vi "Data_Pull_Zmodifiy_Global.vi"(0 "Ceiling":sgl) -> ()   [LabVIEW 2016]
uses:
  Utility/Global Constants.vi
  Utility/Global_Sensor.vi
  Utility/Global_Stage.vi
  Utility/Global_Array.vi
  Program Files/MicroEpsilon/MEDAQLib-3.2.3.19901/Samples/LabView/MEDAQLib/MEDAQLib.lvlib
panel:
  out "Abort Loop":bool
  out "ValueHandle":dbl[](array[numeric])
  in  "block":i32=1
  in  "maxValue":i32=1
  out "avail":i32
  out "Buffer Error":i32
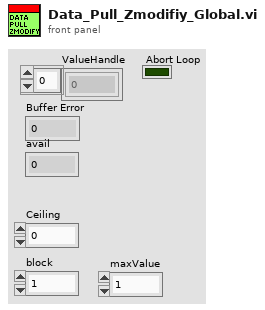
[diagram p1: front panel]
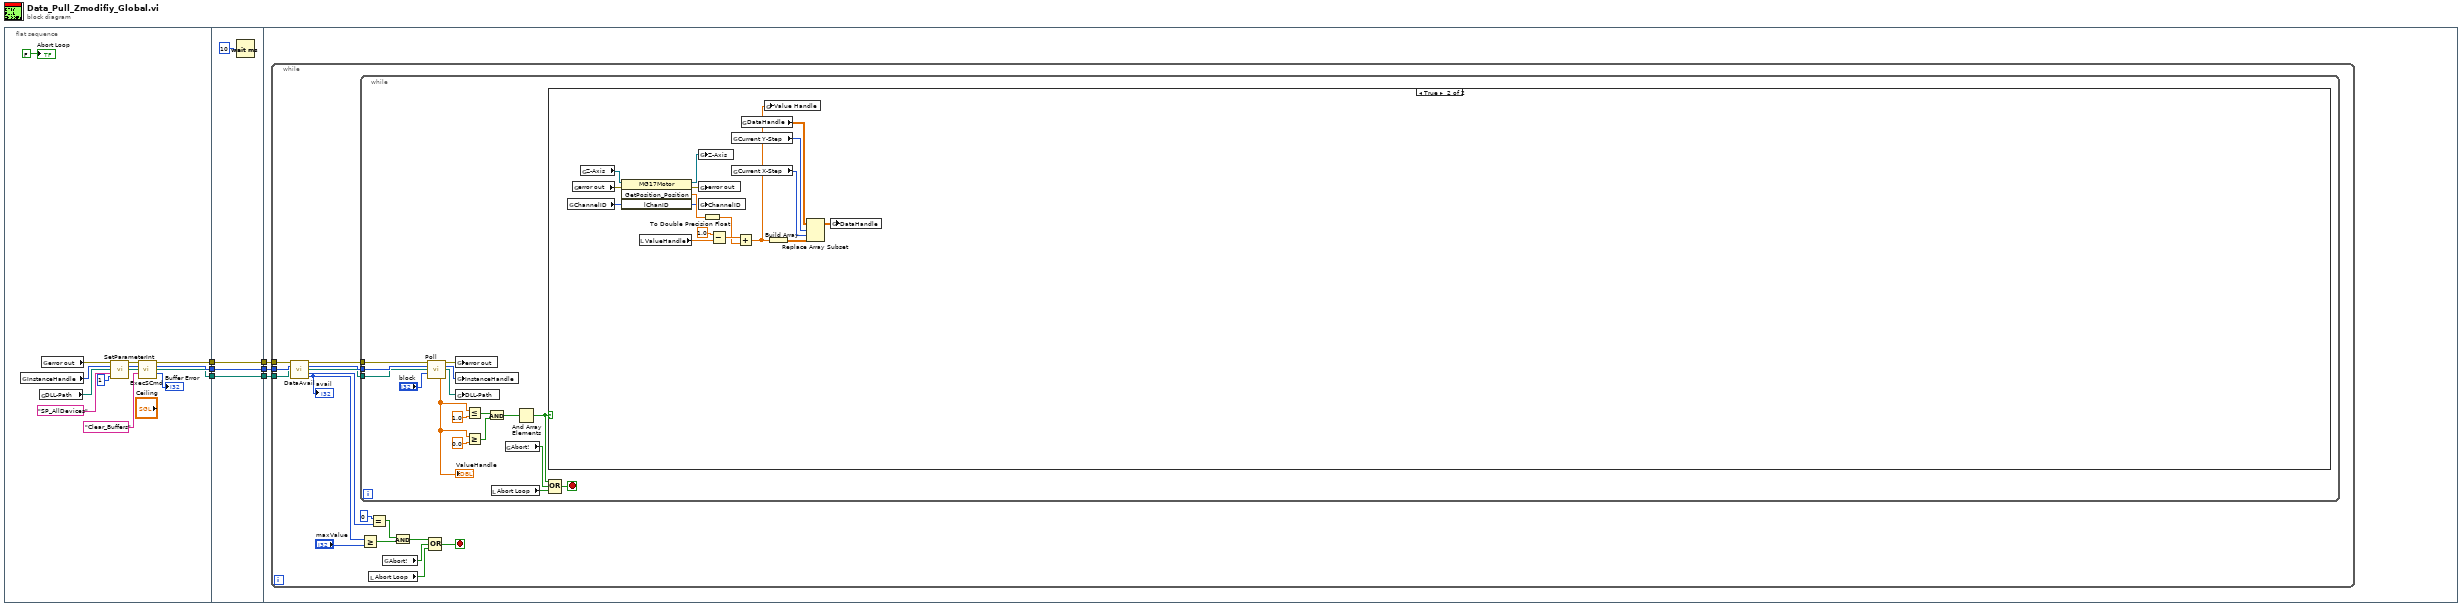
[diagram p0: block diagram]
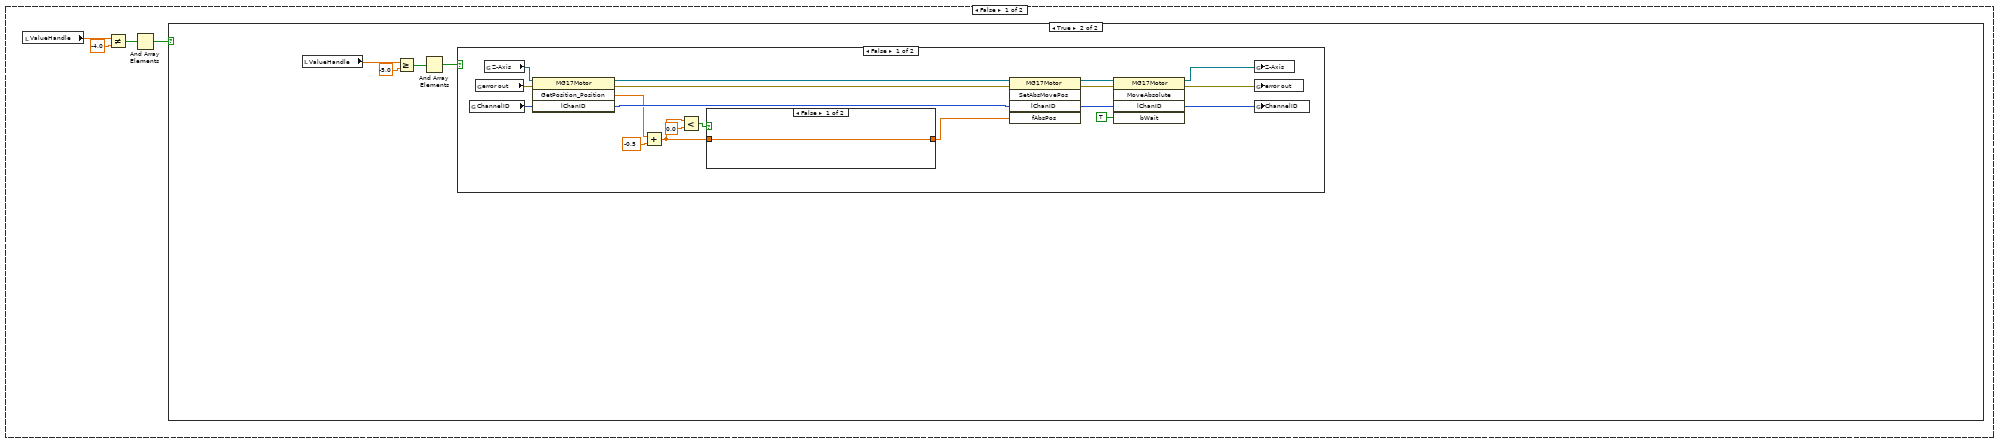
[diagram p2: hidden frame]
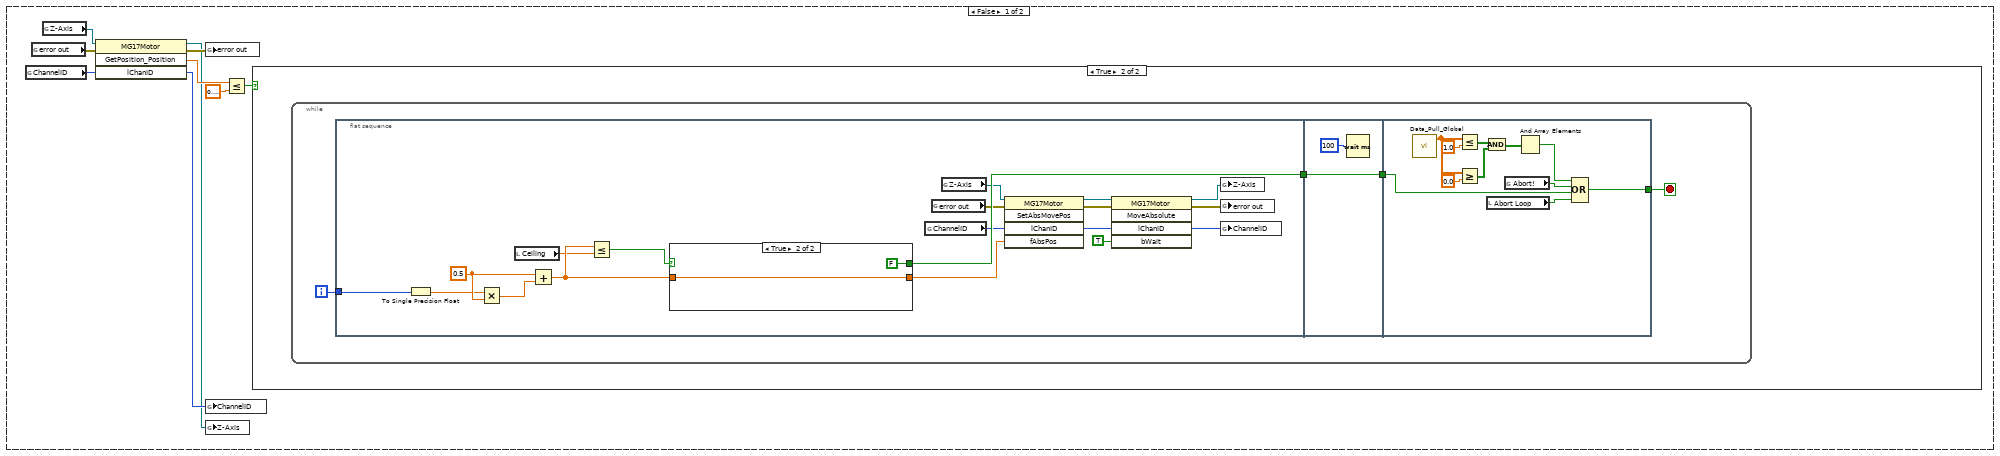
[diagram p3: hidden frame]
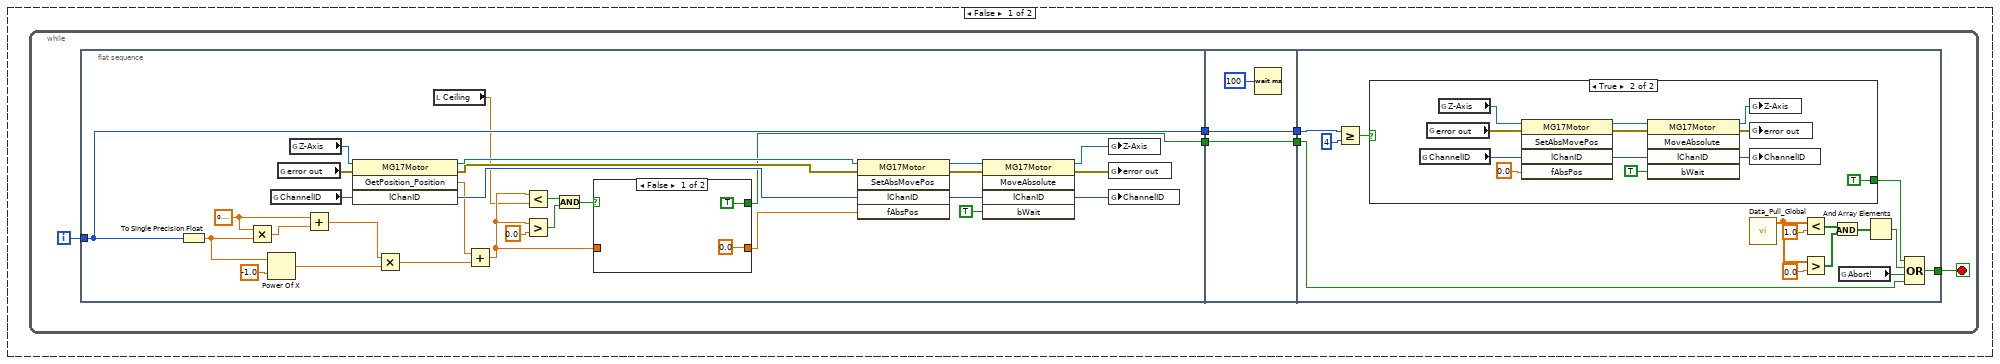
[diagram p4: hidden frame]
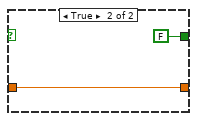
[diagram p5: hidden frame]
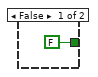
[diagram p6: hidden frame]
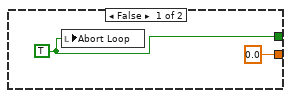
[diagram p7: hidden frame]
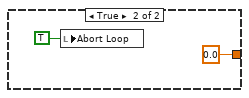
[diagram p8: hidden frame]
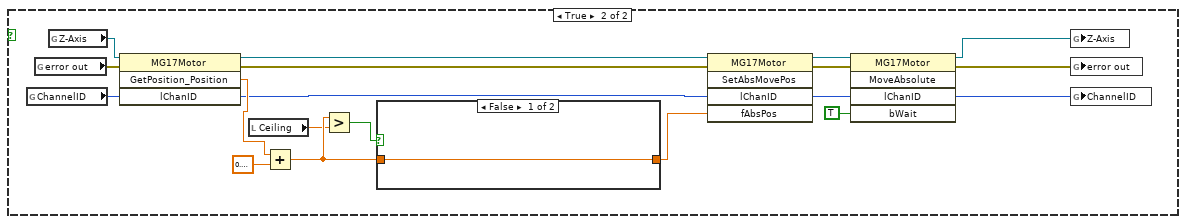
[diagram p9: hidden frame]
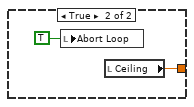
[diagram p10: hidden frame]
diagram:
  n1 = flat-sequence {
    tunnel: [w14] -> w6
    tunnel: [w13] -> w5
    tunnel: [w12] -> w4
    tunnel: [w23] -> w3
    tunnel: w6 -> [w23]
    tunnel: [w22] -> w2
    tunnel: w5 -> [w22]
    tunnel: [w21] -> w1
    tunnel: w4 -> [w21]
    tunnel: w1 -> [w25]
    tunnel: w2 -> [w26]
    tunnel: w3 -> [w27]
    frame #0 {
      n2 = global read "Global_Sensor.vi" "InstanceHandle"() -> (w8:u32)
      n3 = global read "Global_Sensor.vi" "DLL-Path"() -> (w7:path)
      n4 = global read "Global Constants.vi" "error out"() -> (w9:errorcluster)
      n5 = call "SetParameterInt.vi"("Fehler (Eingang, kein Fehler)"=w9, "instanceHandle"=w8, "DLL-Path"=w7, "paramName"="SP_AllDevices", "paramValue"=1) -> ("Fehler (Ausgang)"=w15:errorcluster, "instanceHandle"=w16:u32, "DLL-Path"=w17:path)  [unwired: 7 in, 1 out]
      n6 = call "ExecSCmd.vi"("Fehler (Eingang, kein Fehler)"=w15, "instanceHandle"=w16, "DLL-Path"=w17, "sensorCommand"="Clear_Buffers") -> ("Fehler (Ausgang)"=w14:errorcluster, "instanceHandle"=w13:u32, "DLL-Path"=w12:path, "ERR_CODE"=→"Buffer Error":i32)  [unwired: 8 in]
      "Abort Loop" <- FALSE ("Abort Loop")
    }
    frame #1 {
      n7 = Wait (ms)(milliseconds to wait=u32 10 ("Timer-Wert (ms)")) -> ()  [unwired: 1 out]
    }
    frame #2 {
      n8 = while {
        tunnel: w27 -> [w38]
        tunnel: w26 -> [w37]
        tunnel: w25 -> [w36]
        stop <- w29 stop-if-true
        n9 = call "DataAvail.vi"("Fehler (Eingang, kein Fehler)"=w38, "instanceHandle"=w37, "DLL-Path"=w36) -> ("Fehler (Ausgang)"=w34:errorcluster, "instanceHandle"=w33:u32, "DLL-Path"=w32:path, "ERR_CODE"=w43:i32, "avail"=w41:i32)  [unwired: 8 in]
        "avail" <- w41
        n10 = while {
          tunnel: w34 -> [w59]
          tunnel: w33 -> [w58]
          tunnel: w32 -> [w57]
          stop <- w49 stop-if-true
          n11 = call "Poll.vi"("Fehler (Eingang, kein Fehler)"=w59, "instanceHandle"=w58, "DLL-Path"=w57, "maxValues"="block") -> ("Fehler (Ausgang)"=w47:errorcluster, "instanceHandle"=w45:u32, "DLL-Path"=w44:path, "scaledData"=w51:dbl[])  [unwired: 6 in, 2 out]
          "ValueHandle" <- w51
          n12 = global write "Global Constants.vi" "error out"(w47) -> ()
          n13 = global write "Global_Sensor.vi" "InstanceHandle"(w45) -> ()
          n14 = global write "Global_Sensor.vi" "DLL-Path"(w44) -> ()
          n15 = Less Or Equal?(x=w51, y=1.0 ("Obergrenze")) -> (x <= y?=w54:bool[])
          n16 = Greater Or Equal?(x=w51, y=0.0 ("Untergrenze")) -> (x >= y?=w53:bool[])
          n17 = And(x=w54, y=w53) -> (x .and. y?=w52:bool[])
          n18 = local read "Abort Loop"() -> (w46:bool)
          n19 = global read "Global Constants.vi" "Abort!"() -> (w48:bool)
          n20 = And Array Elements(Boolean array=w52) -> (logical AND=w50:bool)
          n21 = case shown="True" w50 {
            frame False {
              n22 = local read "ValueHandle"() -> (w63:dbl[])
              n23 = Not Equal?(x=w63, y=-4.0) -> (x != y?=w62:bool[])
              n24 = And Array Elements(Boolean array=w62) -> (logical AND=w61:bool)
              n25 = case shown="True" w61 {
                frame False {
                  n26 = global read "Global_Stage.vi" "ChannelID"() -> (w68:i32)
                  n27 = global read "Global Constants.vi" "error out"() -> (w70:errorcluster)
                  n28 = global read "Global_Stage.vi" "Z-Axis"() -> (w66:refnum<k7>)
                  n29 = invoke class="MG17Motor" method="GetPosition_Position"(reference=w66, error in=w70, "lChanID"=w68) -> (reference out=w65:refnum<k7>, error out=w69:errorcluster, "GetPosition_Position"=w71:sgl, "lChanID"=w67:i32)  [unwired: 1 in]
                  n30 = global write "Global Constants.vi" "error out"(w69) -> ()
                  n31 = global write "Global_Stage.vi" "ChannelID"(w67) -> ()
                  n32 = global write "Global_Stage.vi" "Z-Axis"(w65) -> ()
                  n33 = Less Or Equal?(x=w71, y=sgl 0.1) -> (x <= y?=w72:bool)
                  n34 = case shown="True" w72 {
                    frame False {
                      n35 = while {
                        i -> [w79]
                        stop <- w78 stop-if-true
                        n36 = flat-sequence {
                          tunnel: [w88] -> w77
                          tunnel: w79 -> [w87]
                          tunnel: [w87] -> w74
                          tunnel: w77 -> [w115]
                          tunnel: [w115] -> w76
                          tunnel: [w114] -> w75
                          tunnel: w74 -> [w114]
                          tunnel: [w128] -> w78
                          tunnel: w76 -> [w123]
                          tunnel: w75 -> [w122]
                          frame #0 {
                            w105 = sgl 0.4 ("x")
                            n37 = To Single Precision Float(number=w87) -> (single precision float=w106:sgl)
                            n38 = Multiply(x=w105, y=w106) -> (x*y=w104:sgl)
                            n39 = Power Of X(1:sgl -1.0 ("x"), 2:w106) -> (0:w108:sgl)
                            n40 = global read "Global_Stage.vi" "ChannelID"() -> (w81:i32)
                            n41 = global read "Global Constants.vi" "error out"() -> (w85:errorcluster)
                            n42 = global read "Global_Stage.vi" "Z-Axis"() -> (w82:refnum<k7>)
                            n43 = Add(x=w105, y=w104) -> (x+y=w107:sgl)
                            n44 = invoke class="MG17Motor" method="GetPosition_Position"(reference=w82, error in=w85, "lChanID"=w81) -> (reference out=w103:refnum<k7>, error out=w102:errorcluster, "GetPosition_Position"=w99:sgl, "lChanID"=w101:i32)  [unwired: 1 in]
                            n45 = Multiply(x=w107, y=w108) -> (x*y=w100:sgl)
                            n46 = local read "Ceiling"() -> (w80:sgl)
                            n47 = Add(x=w99, y=w100) -> (x+y=w94:sgl)
                            n48 = Less?(x=w94, y=w80) -> (x < y?=w97:bool)
                            n49 = Greater?(x=w94, y=sgl 0.0) -> (0:w96:bool)
                            n50 = And(x=w97, y=w96) -> (x .and. y?=w95:bool)
                            n51 = case shown="False" w95 {
                              tunnel: w94 -> [_ w113]
                              tunnel: [sgl 0.0 w113] -> w93
                              tunnel: [TRUE FALSE] -> w88
                              frame False {
                              }
                              frame True {
                              }
                            }
                            n52 = invoke class="MG17Motor" method="SetAbsMovePos"(reference=w103, error in=w102, "lChanID"=w101, "fAbsPos"=w93) -> (reference out=w92:refnum<k7>, error out=w91:errorcluster, "lChanID"=w90:i32)  [unwired: 1 in, 2 out]
                            n53 = invoke class="MG17Motor" method="MoveAbsolute"(reference=w92, error in=w91, "lChanID"=w90, "bWait"=TRUE) -> (reference out=w84:refnum<k7>, error out=w86:errorcluster, "lChanID"=w83:i32)  [unwired: 1 in, 2 out]
                            n54 = global write "Global_Stage.vi" "Z-Axis"(w84) -> ()
                            n55 = global write "Global Constants.vi" "error out"(w86) -> ()
                            n56 = global write "Global_Stage.vi" "ChannelID"(w83) -> ()
                          }
                          frame #1 {
                            n57 = Wait (ms)(milliseconds to wait=u32 100 ("Zu wartende ms")) -> ()  [unwired: 1 out]
                          }
                          frame #2 {
                            n58 = Greater Or Equal?(x=w122, y=4) -> (x >= y?=w120:bool)
                            n59 = case shown="True" w120 {
                              tunnel: [FALSE TRUE] -> w119
                              frame False {
                              }
                              frame True {
                                n60 = global read "Global_Stage.vi" "ChannelID"() -> (w132:i32)
                                n61 = global read "Global Constants.vi" "error out"() -> (w133:errorcluster)
                                n62 = global read "Global_Stage.vi" "Z-Axis"() -> (w134:refnum<k7>)
                                n63 = invoke class="MG17Motor" method="SetAbsMovePos"(reference=w134, error in=w133, "lChanID"=w132, "fAbsPos"=sgl 0.0) -> (reference out=w142:refnum<k7>, error out=w141:errorcluster, "lChanID"=w140:i32)  [unwired: 1 in, 2 out]
                                n64 = invoke class="MG17Motor" method="MoveAbsolute"(reference=w142, error in=w141, "lChanID"=w140, "bWait"=TRUE) -> (reference out=w137:refnum<k7>, error out=w138:errorcluster, "lChanID"=w136:i32)  [unwired: 1 in, 2 out]
                                n65 = global write "Global_Stage.vi" "Z-Axis"(w137) -> ()
                                n66 = global write "Global Constants.vi" "error out"(w138) -> ()
                                n67 = global write "Global_Stage.vi" "ChannelID"(w136) -> ()
                              }
                            }
                            n68 = call "Data_Pull_Global.vi"() -> ("scaledData"=w117:dbl[])  [unwired: 2 out]
                            n69 = Less?(x=w117, y=1.0) -> (x < y?=w126:bool[])
                            n70 = Greater?(x=w117, y=0.0) -> (0:w125:bool[])
                            n71 = And(x=w126, y=w125) -> (x .and. y?=w124:bool[])
                            n72 = global read "Global Constants.vi" "Abort!"() -> (w118:bool)
                            n73 = And Array Elements(Boolean array=w124) -> (logical AND=w127:bool)
                            n74 = Compound Arithmetic op=OR(w119, w127, w118, w123) -> (w128:bool)
                          }
                        }
                      }
                    }
                    frame True {
                      n75 = while {
                        i -> [w147]
                        stop <- w144 stop-if-true
                        n76 = flat-sequence {
                          tunnel: w147 -> [w165]
                          tunnel: [w155] -> w145
                          tunnel: [w171] -> w146
                          tunnel: w145 -> [w171]
                          tunnel: w146 -> [w177]
                          tunnel: [w176] -> w144
                          frame #0 {
                            w166 = sgl 0.5 ("x")
                            n77 = To Single Precision Float(number=w165) -> (single precision float=w164:sgl)
                            n78 = Multiply(x=w164, y=w166) -> (x*y=w163:sgl)
                            n79 = local read "Ceiling"() -> (w148:sgl)
                            n80 = Add(x=w166, y=w163) -> (x+y=w157:sgl)
                            n81 = Less Or Equal?(x=w157, y=w148) -> (x <= y?=w158:bool)
                            n82 = case shown="True" w158 {
                              tunnel: w157 -> [_ w170]
                              tunnel: [sgl 0.0 w170] -> w156
                              tunnel: [w167 FALSE] -> w155
                              frame False {
                                w167 = TRUE
                                n83 = local write "Abort Loop"(w167) -> ()
                              }
                              frame True {
                              }
                            }
                            n84 = global read "Global_Stage.vi" "ChannelID"() -> (w151:i32)
                            n85 = global read "Global Constants.vi" "error out"() -> (w153:errorcluster)
                            n86 = global read "Global_Stage.vi" "Z-Axis"() -> (w152:refnum<k7>)
                            n87 = invoke class="MG17Motor" method="SetAbsMovePos"(reference=w152, error in=w153, "lChanID"=w151, "fAbsPos"=w156) -> (reference out=w161:refnum<k7>, error out=w162:errorcluster, "lChanID"=w160:i32)  [unwired: 1 in, 2 out]
                            n88 = invoke class="MG17Motor" method="MoveAbsolute"(reference=w161, error in=w162, "lChanID"=w160, "bWait"=TRUE) -> (reference out=w150:refnum<k7>, error out=w154:errorcluster, "lChanID"=w149:i32)  [unwired: 1 in, 2 out]
                            n89 = global write "Global_Stage.vi" "Z-Axis"(w150) -> ()
                            n90 = global write "Global Constants.vi" "error out"(w154) -> ()
                            n91 = global write "Global_Stage.vi" "ChannelID"(w149) -> ()
                          }
                          frame #1 {
                            n92 = Wait (ms)(milliseconds to wait=u32 100 ("Zu wartende ms")) -> ()  [unwired: 1 out]
                          }
                          frame #2 {
                            n93 = call "Data_Pull_Global.vi"() -> ("scaledData"=w173:dbl[])  [unwired: 2 out]
                            n94 = Less Or Equal?(x=w173, y=1.0 ("Obergrenze")) -> (x <= y?=w181:bool[])
                            n95 = Greater Or Equal?(x=w173, y=0.0 ("Untergrenze")) -> (x >= y?=w182:bool[])
                            n96 = And(x=w181, y=w182) -> (x .and. y?=w183:bool[])
                            n97 = local read "Abort Loop"() -> (w174:bool)
                            n98 = global read "Global Constants.vi" "Abort!"() -> (w175:bool)
                            n99 = And Array Elements(Boolean array=w183) -> (logical AND=w178:bool)
                            n100 = Compound Arithmetic op=OR(w178, w175, w177, w174) -> (w176:bool)
                          }
                        }
                      }
                    }
                  }
                }
                frame True {
                  n101 = local read "ValueHandle"() -> (w186:dbl[])
                  n102 = Greater Or Equal?(x=w186, y=-5.0) -> (x >= y?=w184:bool[])
                  n103 = And Array Elements(Boolean array=w184) -> (logical AND=w185:bool)
                  n104 = case shown="False" w185 {
                    frame False {
                      n105 = global read "Global_Stage.vi" "ChannelID"() -> (w189:i32)
                      n106 = global read "Global Constants.vi" "error out"() -> (w201:errorcluster)
                      n107 = global read "Global_Stage.vi" "Z-Axis"() -> (w191:refnum<k7>)
                      n108 = invoke class="MG17Motor" method="GetPosition_Position"(reference=w191, error in=w201, "lChanID"=w189) -> (reference out=w200:refnum<k7>, error out=w199:errorcluster, "GetPosition_Position"=w197:sgl, "lChanID"=w198:i32)  [unwired: 1 in]
                      n109 = Add(x=w197, y=sgl -0.5) -> (x+y=w192:sgl)
                      n110 = Less?(x=w192, y=sgl 0.0) -> (x < y?=w194:bool)
                      n111 = case shown="False" w194 {
                        tunnel: [w207 sgl 0.0] -> w193
                        tunnel: w192 -> [w207 _]
                        frame False {
                        }
                        frame True {
                          n112 = local write "Abort Loop"(TRUE) -> ()
                        }
                      }
                      n113 = invoke on="Methodenknoten" class="MG17Motor" method="SetAbsMovePos"(reference=w200, error in=w199, "lChanID"=w198, "fAbsPos"=w193) -> (reference out=w206:refnum<k7>, error out=w205:errorcluster, "lChanID"=w204:i32)  [unwired: 1 in, 2 out]
                      n114 = invoke on="Methodenknoten" class="MG17Motor" method="MoveAbsolute"(reference=w206, error in=w205, "lChanID"=w204, "bWait"=TRUE) -> (reference out=w190:refnum<k7>, error out=w202:errorcluster, "lChanID"=w188:i32)  [unwired: 1 in, 2 out]
                      n115 = global write "Global_Stage.vi" "Z-Axis"(w190) -> ()
                      n116 = global write "Global Constants.vi" "error out"(w202) -> ()
                      n117 = global write "Global_Stage.vi" "ChannelID"(w188) -> ()
                    }
                    frame True {
                      n118 = global read "Global_Stage.vi" "ChannelID"() -> (w214:i32)
                      n119 = global read "Global Constants.vi" "error out"() -> (w222:errorcluster)
                      n120 = global read "Global_Stage.vi" "Z-Axis"() -> (w212:refnum<k7>)
                      n121 = invoke class="MG17Motor" method="GetPosition_Position"(reference=w212, error in=w222, "lChanID"=w214) -> (reference out=w223:refnum<k7>, error out=w221:errorcluster, "GetPosition_Position"=w218:sgl, "lChanID"=w217:i32)  [unwired: 1 in]
                      n122 = local read "Ceiling"() -> (w211:sgl)
                      n123 = Add(x=w218, y=sgl 0.4) -> (x+y=w216:sgl)
                      n124 = Greater?(x=w216, y=w211) -> (0:w220:bool)
                      n125 = case shown="False" w220 {
                        tunnel: [w229 w230] -> w219
                        tunnel: w216 -> [w229 _]
                        frame False {
                        }
                        frame True {
                          n126 = local write "Abort Loop"(TRUE) -> ()
                          n127 = local read "Ceiling"() -> (w230:sgl)
                        }
                      }
                      n128 = invoke on="Methodenknoten" class="MG17Motor" method="SetAbsMovePos"(reference=w223, error in=w221, "lChanID"=w217, "fAbsPos"=w219) -> (reference out=w228:refnum<k7>, error out=w227:errorcluster, "lChanID"=w225:i32)  [unwired: 1 in, 2 out]
                      n129 = invoke on="Methodenknoten" class="MG17Motor" method="MoveAbsolute"(reference=w228, error in=w227, "lChanID"=w225, "bWait"=TRUE) -> (reference out=w213:refnum<k7>, error out=w224:errorcluster, "lChanID"=w215:i32)  [unwired: 1 in, 2 out]
                      n130 = global write "Global_Stage.vi" "Z-Axis"(w213) -> ()
                      n131 = global write "Global Constants.vi" "error out"(w224) -> ()
                      n132 = global write "Global_Stage.vi" "ChannelID"(w215) -> ()
                    }
                  }
                }
              }
            }
            frame True {
              n133 = global read "Global_Stage.vi" "ChannelID"() -> (w238:i32)
              n134 = global read "Global Constants.vi" "error out"() -> (w244:errorcluster)
              n135 = global read "Global_Stage.vi" "Z-Axis"() -> (w239:refnum<k7>)
              n136 = invoke class="MG17Motor" method="GetPosition_Position"(reference=w239, error in=w244, "lChanID"=w238) -> (reference out=w236:refnum<k7>, error out=w243:errorcluster, "GetPosition_Position"=w248:sgl, "lChanID"=w237:i32)  [unwired: 1 in]
              n137 = local read "ValueHandle"() -> (w246:dbl[])
              n138 = global write "Global_Stage.vi" "Z-Axis"(w236) -> ()
              n139 = global write "Global Constants.vi" "error out"(w243) -> ()
              n140 = global write "Global_Stage.vi" "ChannelID"(w237) -> ()
              n141 = To Double Precision Float(number=w248) -> (double precision float=w234:dbl)
              n142 = Subtract(x=1.0, y=w246) -> (x-y=w245:dbl[])
              n143 = global read "Global Constants.vi" "Current Y-Step"() -> (w242:i32)
              n144 = global read "Global Constants.vi" "Current X-Step"() -> (w232:i32)
              n145 = Add(x=w245, y=w234) -> (x+y=w235:dbl[])
              n146 = global read "Global_Array.vi" "DataHandle"() -> (w240:sgl[][])
              n147 = global write "Global_Array.vi" "Value Handle"(w235) -> ()
              n148 = Build Array(w235) -> (w233:dbl[][])
              n149 = Replace Array Subset(array=w240, new element=w233, index (row)=w242, index (col)=w232) -> (w241:sgl[][])
              n150 = global write "Global_Array.vi" "DataHandle"(w241) -> ()
            }
          }
          n151 = Compound Arithmetic op=OR(w50, w48, w46) -> (w49:bool)
        }
        n152 = Greater Or Equal?(x=w41, y="maxValue") -> (x >= y?=w39:bool)
        n153 = local read "Abort Loop"() -> (w30:bool)
        n154 = Equal?(x=0, y=w43) -> (x = y?=w40:bool)
        n155 = global read "Global Constants.vi" "Abort!"() -> (w28:bool)
        n156 = And(x=w40, y=w39) -> (x .and. y?=w31:bool)
        n157 = Compound Arithmetic op=OR(w31, w28, w30) -> (w29:bool)
      }
    }
  }
